vi "Rinocloud_global_variable.vi"() -> ()   [LabVIEW 2013]
panel:
  in  "Tab Control":enum32{"Communication", "Active items"}(tab)
  in  "Token":string
  in  "Rino url":string="https://rinocloud.com/api/1/files/"
  in  "Local storage root path":path=path "C:/Rinocloud mirror"
  in  "Active item name":string
  in  "Active directory ID":string
  in  "Active file ID":string
  in  "Active object ID":string
  # "These variables need\nto be set by the user."
  # "These variables will be populated by RC_explorer.vi \nThey are meant to improve smooth integration of\nRinocloud library VIs to the custom user's VIs running \non the same machine."
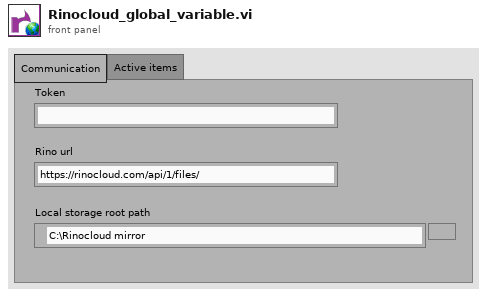
[diagram p1: front panel]
diagram:
